vi "ComplexAlign.vi"(8 "error in (no error)":errorcluster, 11 "Notifiers":T1) -> (0 "error out":errorcluster)   [LabVIEW 2014]
uses:
  support/Notifiers/Notifiers.ctl
  support/Message Handler Loop Notifiers.ctl
  Parameter Analyzer/Parameter Analyzer Notifiers.ctl
  Switching Matrix/Switching Matrix Notifiers.ctl
  Stress Control/StressControl Notifiers.ctl
  Spectrometer/Spectrometer Notifiers.ctl
  Switches and Mirrors/SwitchesMirrors Notifiers.ctl
  Camera/Camera Notifiers.ctl
  XYZ Stage/XYZ Notifications.ctl
  Autofocus Notifiers.ctl
  Measurements/Optoelectronic Measurement/Optoelectronic Notifiers.ctl
  Measurements/Save Data/SaveData Notifiers.ctl
  Measurements/Instrument Sequence/Instrument Sequence Notifiers.ctl
  AutoFocus Functions.ctl
panel:
  # "LICENSED MATERIALS – PROPERTY OF IBM\nCopyright IBM Corp. 2016, 2016\nALL RIGHTS RESERVED"
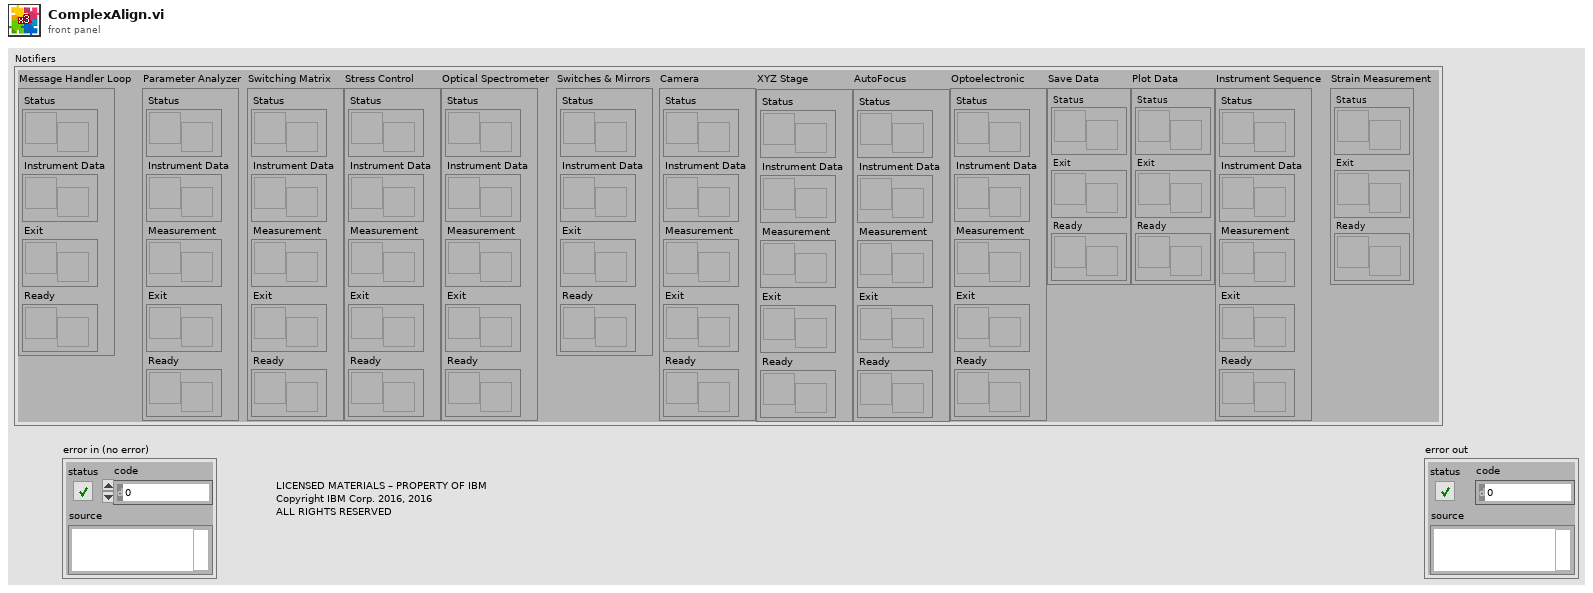
[diagram p1: front panel]
types:
  T1 = typedef "Notifiers.ctl" = cluster{"Message Handler Loop":T2, "Parameter Analyzer":T3, "Switching Matrix":T4, "Stress Control":T5, "Optical Spectrometer":T6, "Switches & Mirrors":T7, "Camera":T8, "XYZ Stage":T9, "AutoFocus":T10, "Optoelectronic":T11, "Save Data":T12, "Plot Data":T12, "Instrument Sequence":T13, "Strain Measurement":cluster{"Status":refnum<notifier>, "Exit":refnum<notifier>, "Ready":refnum<notifier>}}
  T2 = typedef "Message Handler Loop Notifiers.ctl" = cluster{"Status":refnum<notifier>, "Instrument Data":refnum<notifier>, "Exit":refnum<notifier>, "Ready":refnum<notifier>}
  T3 = typedef "Parameter Analyzer Notifiers.ctl" = cluster{"Status":refnum<notifier>, "Instrument Data":refnum<notifier>, "Measurement":refnum<notifier>, "Exit":refnum<notifier>, "Ready":refnum<notifier>}
  T4 = typedef "Switching Matrix Notifiers.ctl" = cluster{"Status":refnum<notifier>, "Instrument Data":refnum<notifier>, "Measurement":refnum<notifier>, "Exit":refnum<notifier>, "Ready":refnum<notifier>}
  T5 = typedef "StressControl Notifiers.ctl" = cluster{"Status":refnum<notifier>, "Instrument Data":refnum<notifier>, "Measurement":refnum<notifier>, "Exit":refnum<notifier>, "Ready":refnum<notifier>}
  T6 = typedef "Spectrometer Notifiers.ctl" = cluster{"Status":refnum<notifier>, "Instrument Data":refnum<notifier>, "Measurement":refnum<notifier>, "Exit":refnum<notifier>, "Ready":refnum<notifier>}
  T7 = typedef "SwitchesMirrors Notifiers.ctl" = cluster{"Status":refnum<notifier>, "Instrument Data":refnum<notifier>, "Exit":refnum<notifier>, "Ready":refnum<notifier>}
  T8 = typedef "Camera Notifiers.ctl" = cluster{"Status":refnum<notifier>, "Instrument Data":refnum<notifier>, "Measurement":refnum<notifier>, "Exit":refnum<notifier>, "Ready":refnum<notifier>}
  T9 = typedef "XYZ Notifications.ctl" = cluster{"Status":refnum<notifier>, "Instrument Data":refnum<notifier>, "Measurement":refnum<notifier>, "Exit":refnum<notifier>, "Ready":refnum<notifier>}
  T10 = typedef "Autofocus Notifiers.ctl" = cluster{"Status":refnum<notifier>, "Instrument Data":refnum<notifier>, "Measurement":refnum<notifier>, "Exit":refnum<notifier>, "Ready":refnum<notifier>}
  T11 = typedef "Optoelectronic Notifiers.ctl" = cluster{"Status":refnum<notifier>, "Instrument Data":refnum<notifier>, "Measurement":refnum<notifier>, "Exit":refnum<notifier>, "Ready":refnum<notifier>}
  T12 = typedef "SaveData Notifiers.ctl" = cluster{"Status":refnum<notifier>, "Exit":refnum<notifier>, "Ready":refnum<notifier>}
  T13 = typedef "Instrument Sequence Notifiers.ctl" = cluster{"Status":refnum<notifier>, "Instrument Data":refnum<notifier>, "Measurement":refnum<notifier>, "Exit":refnum<notifier>, "Ready":refnum<notifier>}
  T14 = typedef "AutoFocus Functions.ctl" = enum16{"Allocate Image Memory", "Free Image Memory", "Grab Image", "Get ROI", "Set ROI", "Set Match Criteria", "Set Target", "Link Stage & Camera", "Set Transformation Matrix", "Find Target", "Align", "Find Focus", "Focus (Gradient)", "Focus (Threshold)", "Focus (Turning Points)", "Update Refnums"}
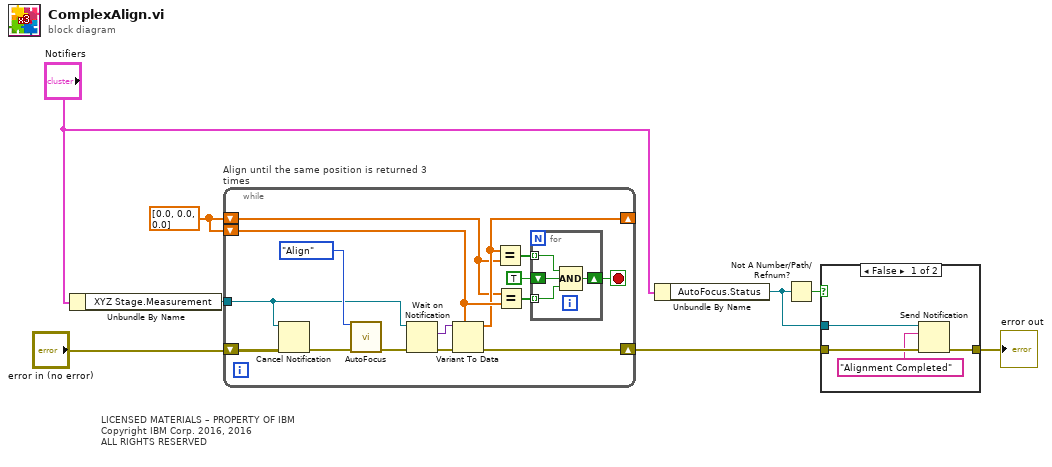
[diagram p0: block diagram]
diagram:
  w6 = dbl[] [0.0, 0.0, 0.0] ("Position")
  # "LICENSED MATERIALS – PROPERTY OF IBM\nCopyright IBM Corp. 2016, 2016\nALL RIGHTS RESERVED"
  n1 = Unbundle By Name("Notifiers") -> ("XYZ Stage.Measurement"=w8:refnum<notifier>)
  n2 = while "Align until the same position is returned 3 times" {
    shift-right: [w12] -> w3
    shift-left: "error in (no error)" -> [w13]
    tunnel: w8 -> [w11]
    shift-right: [w15] -> _
    shift-left: w6 -> [w14]
    shift-left: w6 -> [w18]
    stop <- w20 stop-if-true
    n3 = Cancel Notification(0:w11, 3:w13) -> (11:w9:errorcluster)  [unwired: 2 out]
    n4 = call "AutoFocus.vi"("Function"=AutoFocus_Functions."Align", "error in (no error)"=w9) -> ("error out"=w10:errorcluster)  [unwired: 10 in, 3 out]
    n5 = Wait on Notification(notifier=w11, error in (no error)=w10) -> (notification=w22:variant, error out=w23:errorcluster)  [unwired: 4 out]
    n6 = Variant To Data(error in=w23, type=w18, Variant=w22) -> (data=w15:dbl[], error out=w12:errorcluster)
    n7 = Equal?(x=w15, y=w14) -> (x = y?=w17:bool[])
    n8 = Equal?(x=w14, y=w18) -> (x = y?=w16:bool[])
    n9 = for {
      tunnel: w17 -> [w24] mode=indexing
      shift-right: [w26] -> w20
      shift-left: TRUE -> [w25]
      tunnel: w16 -> [w27] mode=indexing
      n10 = Compound Arithmetic op=AND(w24, w25, w27) -> (w26:bool)
    }
  }
  n11 = Unbundle By Name("Notifiers") -> ("AutoFocus.Status"=w4:refnum<notifier>)
  n12 = Not A Number/Path/Refnum?(number/path/refnum=w4) -> (NaN/Path/Refnum?=w5:bool)
  n13 = case shown="False" w5 {
    tunnel: w3 -> [w31 w32]
    tunnel: [w30 w32] -> w2
    tunnel: w4 -> [w29 _]
    frame False {
      n14 = Send Notification(notification="Alignment Completed", notifier=w29, error in (no error)=w31) -> (error out=w30:errorcluster)  [unwired: 1 out]
    }
    frame True {
    }
  }
  "error out" <- w2
